vi "Write Report.vi"(8 "error in (no error)":errorcluster, 10 "Resource In":variant, 11 "Analyze Parameter Energy in":refnum<class "Analyze Parameter Energy.lvclass">) -> (0 "error out":errorcluster, 2 "Resource Out":variant, 3 "Analyze Parameter Energy out":refnum<class "Analyze Parameter Energy.lvclass">)   [LabVIEW 2020, in "Analyze Parameter Energy.lvclass"]
uses:
  Analyze Parameter Energy.lvclass
  C:/POLARIS Programme/POLARIS-AS-3-Cams/Submodules/HIJ Vision/Analyze/Analyze Parameter/Analyze Parameter Base/Analyze Parameter Base.lvclass
  <vilib>/Utility/config.llb/Config Data RefNum.ctl
  Analyze Parameter Energy.lvclass/Analyze Parameter Energy.ctl
  Read Energy.vi
  <vilib>/Utility/config.llb/Write Key (Double).vi
  <vilib>/Utility/config.llb/NI_LVConfig.lvlib
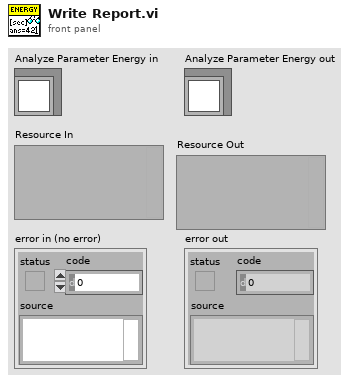
[diagram p1: front panel]
types:
  T1 = typedef "NI_LVConfig.lvlib/Config Data RefNum.ctl" = refnum<k1>
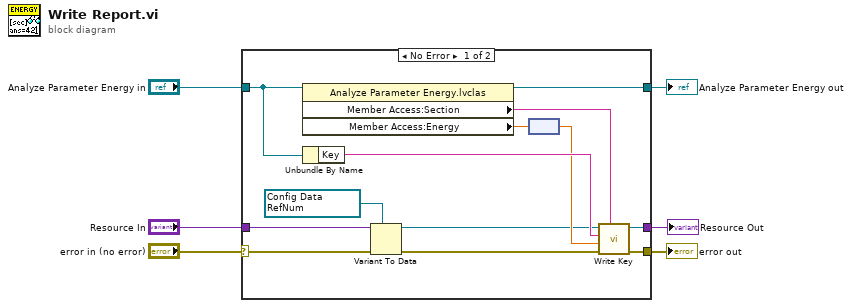
[diagram p0: block diagram]
diagram:
  n1 = case shown="No Error" "error in (no error)" {
    selector: "error in (no error)" -> [w10 w21]
    tunnel: "Analyze Parameter Energy in" -> [w7 w20]
    tunnel: [w13 w20] -> w2
    tunnel: [w15 w22] -> w4
    tunnel: [w14 w21] -> w3
    tunnel: "Resource In" -> [w12 w22]
    frame No Error {
      w8 = T1 refnum items=["config data"] ("refnum")
      n2 = property class="Analyze Parameter Energy.lvclas"(reference=w7) -> (reference out=w13:refnum<class "Analyze Parameter Energy.lvclass">, "Member Access:Section"=w17:string, "Member Access:Energy"=w18:dbl[unit])  [unwired: 1 in, 1 out]
      n3 = Unbundle By Name(w7) -> ("Key"=w19:string)
      n4 = Variant To Data(error in=w10, type=w8, Variant=w12) -> (data=w11:T1, error out=w9:errorcluster)
      n5 = node(w18) -> (w16:dbl)
      n6 = call-poly <vilib>:"Write Key.vi"("section"=w17, "error in (no error)"=w9, "value"=w16, "key"=w19, "refnum"=w11) -> ("error out"=w14:errorcluster, "refnum out"=w15:T1)  [unwired: 4 in, 1 out]
    }
    frame Error {
    }
  }
  "error out" <- w3
  "Analyze Parameter Energy out" <- w2
  "Resource Out" <- w4
